vi "zero top.vi"(7 "zero":bool, 8 "Stepper 0 error in":errorcluster, 9 "Stepper 0 in":T1, 10 "Pin 2 error in":errorcluster, 11 "Pin 2 in":T1) -> (0 "Stepper 0 error out":errorcluster, 1 "Stepper 0 out":T1, 2 "Pin 2 error out":errorcluster, 3 "Pin 2 out":T1)   [LabVIEW 2018]
uses:
  <vilib>/LabVIEW Interface for Arduino/Type Defs/Arduino Resource.ctl
  <vilib>/LabVIEW Interface for Arduino/Type Defs/Board Type.ctl
  Control 1a.ctl
  <vilib>/LabVIEW Interface for Arduino/LabVIEW Interface for Arduino.lvlib
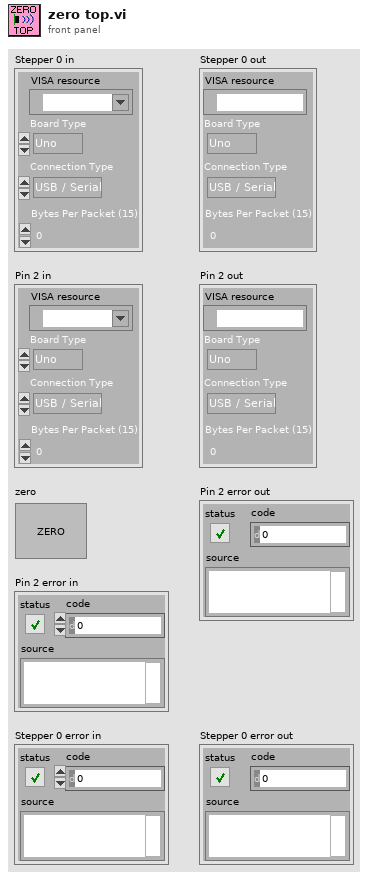
[diagram p1: front panel]
types:
  T1 = typedef "LabVIEW Interface for Arduino.lvlib/Arduino Resource.ctl" = cluster{"VISA resource":refnum<visa-resource-name>, "Board Type":T2, "Connection Type":enum8{"USB / Serial"}, "Bytes Per Packet (15)":u8}
  T2 = typedef "LabVIEW Interface for Arduino.lvlib/Board Type.ctl" = enum16{"Uno", "Dimuelanove w/Atmega 328", "Mega 2560"}
  T3 = typedef "Control 1a.ctl" = enum16{"initialize", "stage 1", "stage 2", "stage 3", "stage 4", "stage 5", "close"}
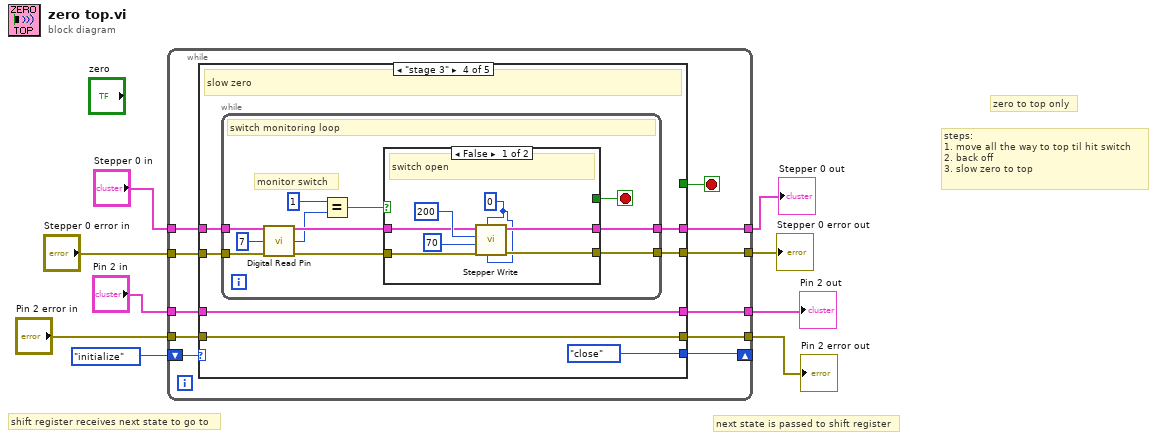
[diagram p0: block diagram]
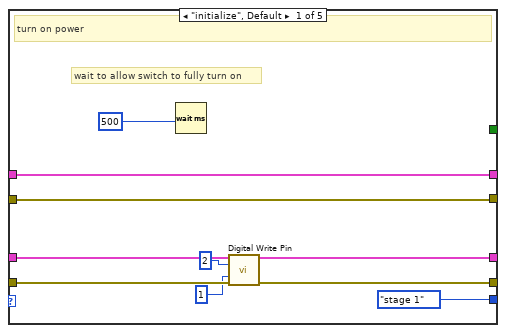
[diagram p2: hidden frame]
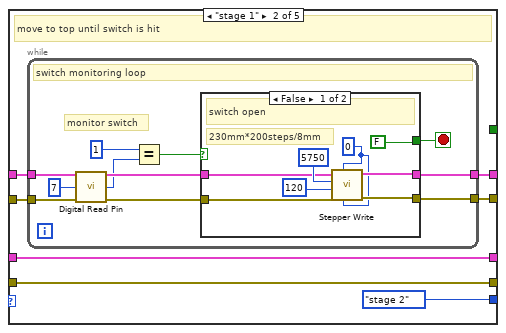
[diagram p3: hidden frame]
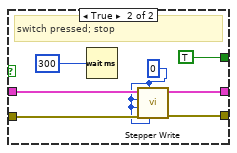
[diagram p4: hidden frame]
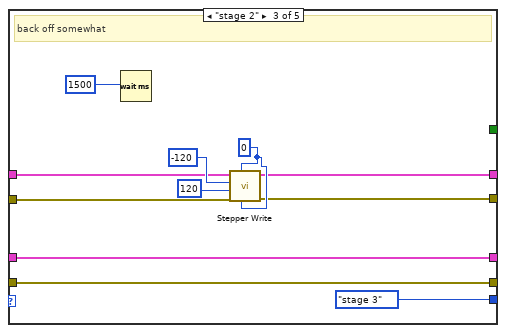
[diagram p5: hidden frame]
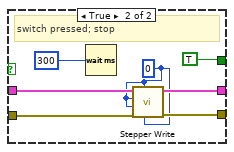
[diagram p6: hidden frame]
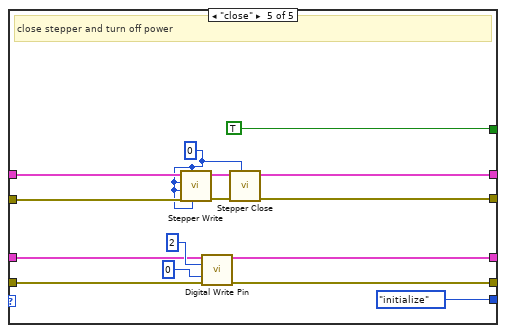
[diagram p7: hidden frame]
diagram:
  # "steps:\n1. move all the way to top til hit switch\n2. back off\n3. slow zero to top"
  # "zero to top only"
  # "shift register receives next state to go to"
  # "next state is passed to shift register"
  n1 = while {
    shift-right: [w17] -> _
    shift-left: Control_1a."initialize" -> [w20]
    tunnel: "Stepper 0 in" -> [w19]
    tunnel: "Stepper 0 error in" -> [w18]
    tunnel: [w15] -> w5
    tunnel: [w14] -> w6
    tunnel: [w13] -> w7
    tunnel: [w12] -> w1
    tunnel: "Pin 2 in" -> [w11]
    tunnel: "Pin 2 error in" -> [w10]
    stop <- w16 stop-if-true
    n2 = case shown="\"stage 3\"" w20 {
      tunnel: w19 -> [w29 w34 w68 w80 w119]
      tunnel: w18 -> [w28 w33 w67 w79 w118]
      tunnel: [w28 w31 w65 w77 w110] -> w14
      tunnel: [w29 w32 w66 w78 w111] -> w15
      tunnel: [Control_1a."stage 1" Control_1a."stage 2" Control_1a."stage 3" Control_1a."close" Control_1a."initialize"] -> w17
      tunnel: [_ _ _ _ TRUE] -> w16
      tunnel: [w25 w36 w74 w76 w115] -> w13
      tunnel: [w24 w35 w73 w75 w114] -> w12
      tunnel: w11 -> [w23 w36 w74 w76 w113]
      tunnel: w10 -> [w22 w35 w73 w75 w112]
      frame "initialize", Default {
        # "wait to allow switch to fully turn on"
        # "turn on power"
        n3 = Wait (ms)(milliseconds to wait=500) -> ()  [unwired: 1 out]
        n4 = call <vilib>:"Digital Write Pin.vi"("Arduino Resource"=w23, "Digital I/O Pin (0)"=2, "Value (0)"=1, "error in"=w22) -> ("Arduino Resource"=w25:T1, "error out"=w24:errorcluster)  [unwired: 10 in]
      }
      frame "stage 1" {
        # "move to top until switch is hit"
        n5 = while {
          tunnel: w34 -> [w46]
          tunnel: w33 -> [w45]
          tunnel: [w42] -> w32
          tunnel: [w41] -> w31
          stop <- w47 stop-if-true
          # "monitor switch"
          # "switch monitoring loop"
          n6 = call <vilib>:"Digital Read Pin.vi"("Arduino Resource"=w46, "Digital I/O Pin (0)"=7, "error in"=w45) -> ("Arduino Resource"=w44:T1, "Value"=w38:u8, "error out"=w43:errorcluster)  [unwired: 10 in]
          n7 = Equal?(x=1, y=w38) -> (x = y?=w40:bool)
          n8 = case shown="False" w40 {
            tunnel: [FALSE TRUE] -> w47
            tunnel: w44 -> [w54 w62]
            tunnel: w43 -> [w52 w61]
            tunnel: [w53 w60] -> w42
            tunnel: [w51 w59] -> w41
            frame False {
              w50 = 0
              # "230mm*200steps/8mm"
              # "switch open"
              n9 = call <vilib>:"Stepper Write.vi"("Set Acceleration (0 to disable)"=w50, "Stepper #"=w50, "error in"=w52, "Set Speed (Steps per Second)"=120, "# of Steps to Move"=5750, "Arduino Resource"=w54) -> ("error out"=w51:errorcluster, "Arduino Resource Out"=w53:T1)  [unwired: 4 in]
            }
            frame True {
              w57 = 0
              # "switch pressed; stop"
              n10 = Wait (ms)(milliseconds to wait=300) -> ()  [unwired: 1 out]
              n11 = call <vilib>:"Stepper Write.vi"("Set Acceleration (0 to disable)"=w57, "Stepper #"=w57, "error in"=w61, "Set Speed (Steps per Second)"=w57, "# of Steps to Move"=w57, "Arduino Resource"=w62) -> ("error out"=w59:errorcluster, "Arduino Resource Out"=w60:T1)  [unwired: 4 in]
            }
          }
        }
      }
      frame "stage 2" {
        w69 = 0
        # "back off somewhat"
        n12 = Wait (ms)(milliseconds to wait=1500) -> ()  [unwired: 1 out]
        n13 = call <vilib>:"Stepper Write.vi"("Set Acceleration (0 to disable)"=w69, "Stepper #"=w69, "error in"=w67, "Set Speed (Steps per Second)"=120, "# of Steps to Move"=-120, "Arduino Resource"=w68) -> ("error out"=w65:errorcluster, "Arduino Resource Out"=w66:T1)  [unwired: 4 in]
      }
      frame "stage 3" {
        # "slow zero"
        n14 = while {
          tunnel: w80 -> [w90]
          tunnel: w79 -> [w89]
          tunnel: [w86] -> w78
          tunnel: [w85] -> w77
          stop <- w91 stop-if-true
          # "monitor switch"
          # "switch monitoring loop"
          n15 = call <vilib>:"Digital Read Pin.vi"("Arduino Resource"=w90, "Digital I/O Pin (0)"=7, "error in"=w89) -> ("Arduino Resource"=w88:T1, "Value"=w82:u8, "error out"=w87:errorcluster)  [unwired: 10 in]
          n16 = Equal?(x=1, y=w82) -> (x = y?=w84:bool)
          n17 = case shown="False" w84 {
            tunnel: [_ TRUE] -> w91
            tunnel: w88 -> [w97 w105]
            tunnel: w87 -> [w95 w104]
            tunnel: [w96 w103] -> w86
            tunnel: [w94 w102] -> w85
            frame False {
              w93 = 0
              # "switch open"
              n18 = call <vilib>:"Stepper Write.vi"("Set Acceleration (0 to disable)"=w93, "Stepper #"=w93, "error in"=w95, "Set Speed (Steps per Second)"=70, "# of Steps to Move"=200, "Arduino Resource"=w97) -> ("error out"=w94:errorcluster, "Arduino Resource Out"=w96:T1)  [unwired: 4 in]
            }
            frame True {
              w100 = 0
              # "switch pressed; stop"
              n19 = Wait (ms)(milliseconds to wait=300) -> ()  [unwired: 1 out]
              n20 = call <vilib>:"Stepper Write.vi"("Set Acceleration (0 to disable)"=w100, "Stepper #"=w100, "error in"=w104, "Set Speed (Steps per Second)"=w100, "# of Steps to Move"=w100, "Arduino Resource"=w105) -> ("error out"=w102:errorcluster, "Arduino Resource Out"=w103:T1)  [unwired: 4 in]
            }
          }
        }
      }
      frame "close" {
        w107 = 0
        # "close stepper and turn off power"
        n21 = call <vilib>:"Stepper Write.vi"("Set Acceleration (0 to disable)"=w107, "Stepper #"=w107, "error in"=w118, "Set Speed (Steps per Second)"=w107, "# of Steps to Move"=w107, "Arduino Resource"=w119) -> ("error out"=w108:errorcluster, "Arduino Resource Out"=w109:T1)  [unwired: 4 in]
        n22 = call <vilib>:"Digital Write Pin.vi"("Arduino Resource"=w113, "Digital I/O Pin (0)"=2, "Value (0)"=0, "error in"=w112) -> ("Arduino Resource"=w115:T1, "error out"=w114:errorcluster)  [unwired: 10 in]
        n23 = call <vilib>:"Stepper Close.vi"("Stepper #"=w107, "error in"=w108, "Arduino Resource"=w109) -> ("error out"=w110:errorcluster, "Arduino Resource Out"=w111:T1)  [unwired: 7 in]
      }
    }
  }
  "Pin 2 error out" <- w1
  "Pin 2 out" <- w7
  "Stepper 0 error out" <- w6
  "Stepper 0 out" <- w5
